vi "Configure VIPC Apply.vi"(8 "error in (no error)":errorcluster, 10 "JSON string":string) -> (0 "error out":errorcluster, 3 "VIPC Apply out":refnum<class "VIPC Apply.lvclass">)   [LabVIEW 2014, in "VIPC Apply.lvclass"]
uses:
  VIPC Apply.lvclass
  VIPC Apply - STYP.ctl
  VIPC Apply.lvclass/VIPC Apply.ctl
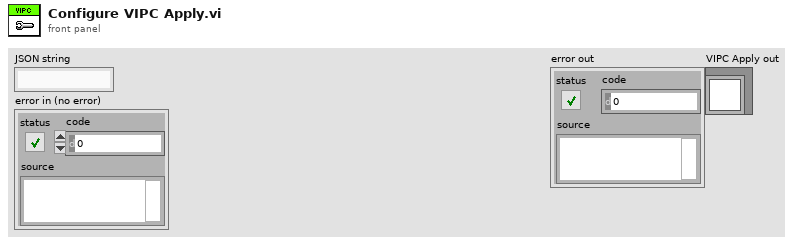
[diagram p1: front panel]
types:
  T1 = typedef "VIPC Apply - STYP.ctl" = cluster{"VIPC Path":string, "LabVIEW Version":string}
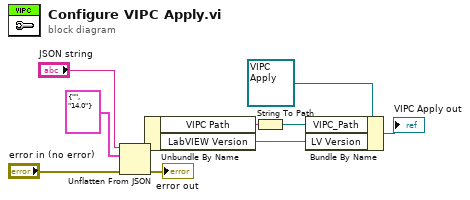
[diagram p0: block diagram]
diagram:
  n1 = Unflatten From JSON(JSON string="JSON string", type and defaults=T1 {"VIPC Path"="", "LabVIEW Version"="14.0"} ("VIPC Apply"), error in (no error)="error in (no error)") -> (value=w6:T1, error out=→"error out":errorcluster)  [unwired: 4 in]
  n2 = Unbundle By Name(w6) -> ("VIPC Path"=w4:string, "LabVIEW Version"=w1:string)
  n3 = String To Path(string=w4) -> (path=w3:path)
  n4 = Bundle By Name(cluster=refnum<class "VIPC Apply.lvclass"> refnum ("VIPB Build out"), "VIPC_Path"=w3, "LV Version"=w1) -> (→"VIPC Apply out":refnum<class "VIPC Apply.lvclass">)
